vi "Populate Device Names Listbox.vi"(0 "LstBox Refnum":refnum<vi>, 1 "client handle":T1, 2 "XML File Path":path, 3 "error in (no error)":errorcluster) -> (5 "ACNET Devices out":refnum<class "ACNET Devices.lvclass">, 6 "XML File Path (duplicate)":path, 7 "error out":errorcluster)   [LabVIEW 2013, in "ACNET Monitor.lvlib"]
uses:
  ACNET Monitor.lvlib
  ACNET Devices.lvclass
  <vilib>/httpClient/ClientHandle.ctl
  ACNET Device.lvclass
  <vilib>/httpClient/LabVIEWHTTPClient.lvlib
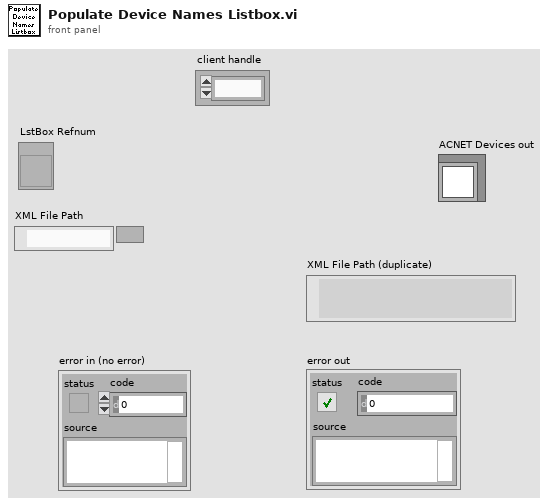
[diagram p1: front panel]
types:
  T1 = typedef "LabVIEWHTTPClient.lvlib/ClientHandle.ctl" = refnum<k1>
  T2 = cluster{"Name":string, "Units":string, "Value":string}[]
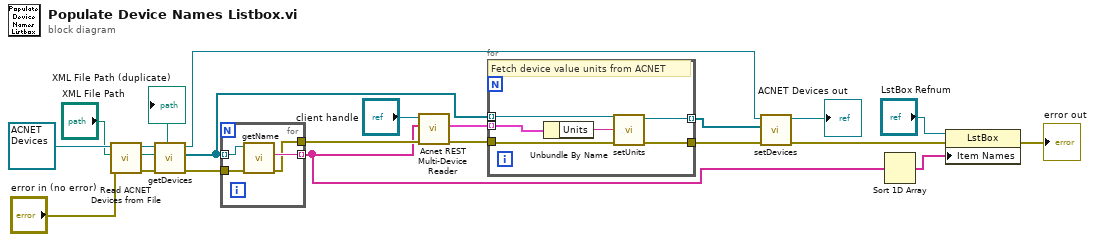
[diagram p0: block diagram]
diagram:
  n1 = call "Read ACNET Devices from File.vi"("error in (no error)"="error in (no error)", "XML File Path"="XML File Path", "ACNET Devices in"=refnum<class "ACNET Devices.lvclass"> refnum ("ACNET Device Limits List in")) -> ("error out"=w20:errorcluster, "XML File Path (duplicate)"=→"XML File Path (duplicate)":path, "ACNET Devices out"=w19:refnum<class "ACNET Devices.lvclass">)  [unwired: 6 in]
  n2 = call-dynamic "getDevices.vi"("error in (no error)"=w20, "ACNET Devices in"=w19) -> ("error out"=w21:errorcluster, "Devices"=w10:refnum<class "ACNET Device.lvclass">[], "ACNET Devices out"=w7:refnum<class "ACNET Devices.lvclass">)  [unwired: 7 in]
  n3 = for {
    tunnel: w10 -> [w24] mode=indexing
    tunnel: w21 -> [w25]
    tunnel: [w23] -> w1 mode=indexing
    tunnel: [w22] -> w11
    n4 = call-dynamic "getName.vi"("error in (no error)"=w25, "ACNET Device in"=w24) -> ("error out"=w22:errorcluster, "name"=w23:string)  [unwired: 7 in, 1 out]
  }
  n5 = call "Acnet REST Multi-Device Reader.vi"("error in (no error)"=w11, "Devices"=w1, "client handle"="client handle") -> ("error out"=w8:errorcluster, "ACNET Device Readings"=w9:T2)  [unwired: 6 in, 1 out]
  n6 = for {
    tunnel: w10 -> [w31] mode=indexing
    tunnel: w9 -> [w30] mode=indexing
    tunnel: w8 -> [w28]
    tunnel: [w27] -> w4
    tunnel: [w26] -> w6 mode=indexing
    # "Fetch device value units from ACNET"
    n7 = Unbundle By Name(w30) -> ("Units"=w29:string)
    n8 = call-dynamic "setUnits.vi"("error in (no error)"=w28, "units"=w29, "ACNET Device in"=w31) -> ("error out"=w27:errorcluster, "ACNET Device out"=w26:refnum<class "ACNET Device.lvclass">)  [unwired: 7 in]
  }
  n9 = call-dynamic "setDevices.vi"("error in (no error)"=w4, "Devices"=w6, "ACNET Devices in"=w7) -> ("error out"=w3:errorcluster, "ACNET Devices out"=→"ACNET Devices out":refnum<class "ACNET Devices.lvclass">)  [unwired: 7 in]
  n10 = Sort 1D Array(array=w1) -> (sorted array=w2:string[])
  n11 = property on="Property Node" class="LstBox"(reference="LstBox Refnum", error in=w3, "Item Names"=w2) -> (error out=→"error out":errorcluster)  [unwired: 1 out]
